vi "Initialize.vi"(8 "error in (no error)":errorcluster) -> (0 "error out":errorcluster, 2 "User Event Out":refnum<event-registration>, 3 "queue out":refnum<queue>)   [LabVIEW 2018, in "Queue Library.lvlib"]
uses:
  Queue Library.lvlib
  Controls/Message.ctl
  Controls/State.ctl
  User Event Action Enum.ctl
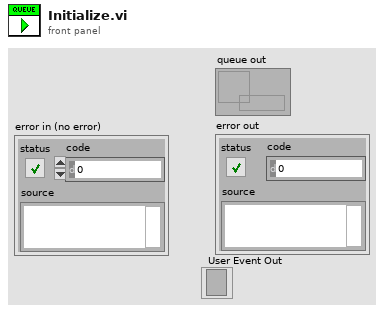
[diagram p1: front panel]
types:
  T1 = typedef "Queue Library.lvlib/User Event Action Enum.ctl" = enum16{"Initialize", "Generate", "Destroy"}
  T2 = typedef "State.ctl" = enum16{"Initialize", "Idle", "Start Scope", "Acquire", "Stop Scope", "Config FGen", "Start FGen", "Sweep FGen", "Stop FGen", "Plot", "Option Selection", "Channel 0 Selection", "Channel 1 Selection", "Update Cursors", "Update Measurements", "Time/Div", "Autoscale", "Stop", "Error"}
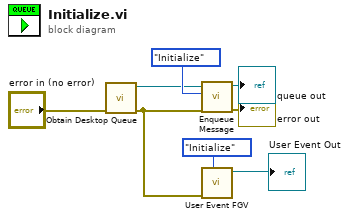
[diagram p0: block diagram]
diagram:
  n1 = call "Obtain Desktop Queue.vi"("error in (no error)"="error in (no error)") -> ("error out"=w3:errorcluster, "queue out"=w7:refnum<queue>)  [unwired: 9 in]
  n2 = call "Enqueue Message.vi"("error in (no error)"=w3, "State"=State."Initialize", "queue in"=w7) -> ("error out"=→"error out":errorcluster, "queue out"=→"queue out":refnum<queue>)  [unwired: 7 in]
  n3 = call "User Event FGV.vi"("Action"=User_Event_Action_Enum."Initialize", "error in (no error)"=w3) -> ("Event Registration Refnum out"=→"User Event Out":refnum<event-registration>)  [unwired: 8 in, 1 out]
